vi "Parse Pattern Name.vi"(8 "error in (no error)":errorcluster, 10 "Index":i32, 11 "Pattern Name":string) -> (0 "error out":errorcluster, 3 "Pattern Name out":string)   [LabVIEW 2018, in "File Parser Interface.lvlib" / "File Parser Interface.lvclass"]
uses:
  File Parser Interface.lvclass
  Operations - FGV.ctl
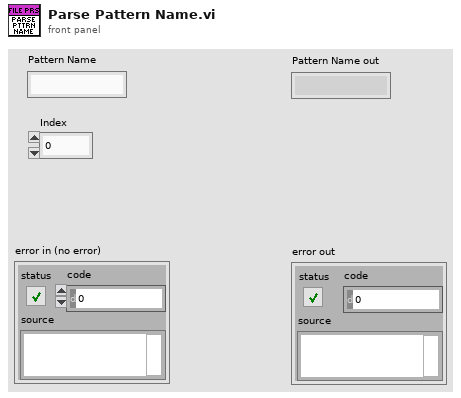
[diagram p1: front panel]
types:
  T1 = typedef "File Parser Interface.lvlib/File Parser Interface.lvclass/Operations - FGV.ctl" = enum16{"Set", "Get", "Clear"}
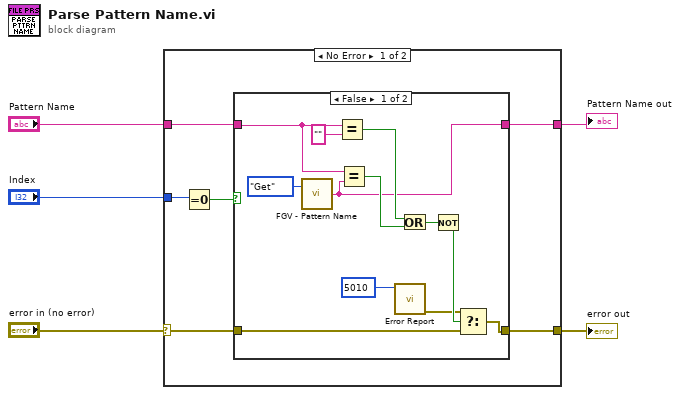
[diagram p0: block diagram]
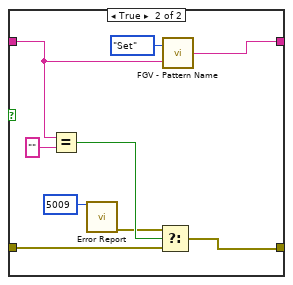
[diagram p2: hidden frame]
diagram:
  n1 = case shown="No Error" "error in (no error)" {
    selector: "error in (no error)" -> [w7 w33]
    tunnel: "Pattern Name" -> [w9 w34]
    tunnel: "Index" -> [w11 _]
    tunnel: [w6 w33] -> w2
    tunnel: [w8 w34] -> w1
    frame No Error {
      n2 = Equal To 0?(x=w11) -> (x = 0?=w10:bool)
      n3 = case shown="False" w10 {
        tunnel: w9 -> [w16 w27]
        tunnel: [w12 w26] -> w8
        tunnel: w7 -> [w20 w30]
        tunnel: [w19 w29] -> w6
        frame False {
          n4 = call "FGV - Pattern Name.vi"("Operation"=Operations_-_FGV."Get") -> ("String out"=w12:string)  [unwired: 1 in]
          n5 = Equal?(x=w16, y="") -> (x = y?=w22:bool)
          n6 = Equal?(x=w16, y=w12) -> (x = y?=w21:bool)
          n7 = call "Error Report.vi"("Error Code"=i16 5010) -> ("error out"=w13:errorcluster)  [unwired: 10 in]
          n8 = Or(x=w22, y=w21) -> (x .or. y?=w18:bool)
          n9 = Not(x=w18) -> (.not. x?=w17:bool)
          n10 = Select(t=w13, s=w17, f=w20) -> (s? t:f=w19:errorcluster)
        }
        frame True {
          n11 = Equal?(x=w27, y="") -> (x = y?=w31:bool)
          n12 = call "Error Report.vi"("Error Code"=i16 5009) -> ("error out"=w24:errorcluster)  [unwired: 10 in]
          n13 = Select(t=w24, s=w31, f=w30) -> (s? t:f=w29:errorcluster)
          n14 = call "FGV - Pattern Name.vi"("String"=w27, "Operation"=Operations_-_FGV."Set") -> ("String out"=w26:string)
        }
      }
    }
    frame Error {
    }
  }
  "Pattern Name out" <- w1
  "error out" <- w2
